vi "GenerateDefaultIBWFile.vi"(8 "error in (no error)":errorcluster) -> (0 "error out":errorcluster, 3 "Path":path)   [LabVIEW 2019]
uses:
  <vilib>/Utility/sysdir.llb/Get System Directory.vi
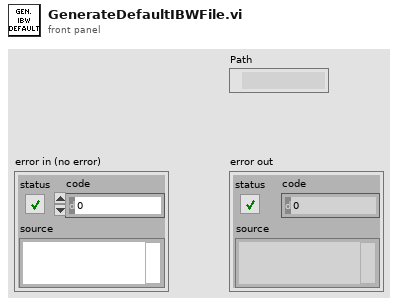
[diagram p1: front panel]
types:
  T1 = enum16{"open", "replace", "create", "open or create", "replace or create", "replace or create with confirmation"}
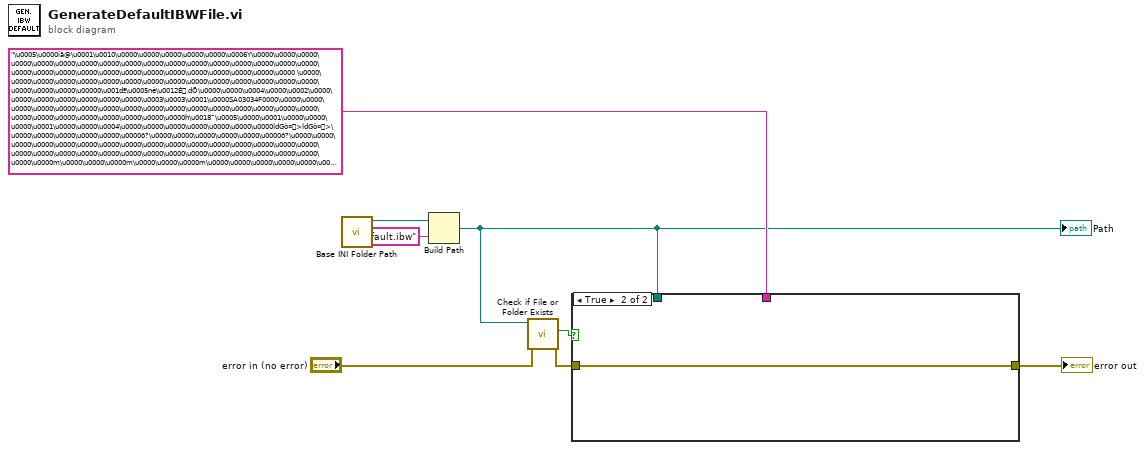
[diagram p0: block diagram]
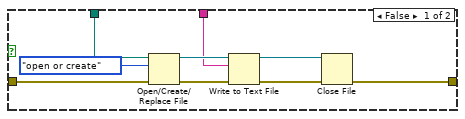
[diagram p2: hidden frame]
diagram:
  n1 = call "Base INI Folder Path.vi"() -> ("Base Path"=w8:path)  [unwired: 11 in]
  n2 = Build Path(base path=w8, name or relative path="Default.ibw") -> (appended path=w1:path)
  "Path" <- w1
  n3 = call <vilib>:"Check if File or Folder Exists.vi"("error in (no error)"="error in (no error)", "path"=w1) -> ("error out"=w3:errorcluster, "file or folder exists?"=w2:bool)  [unwired: 7 in, 1 out]
  n4 = case shown="True" w2 {
    tunnel: w1 -> [w17 _]
    tunnel: "\u0005\u0000îä@\u0001\u0010\u0000\u0000\u0000\u0000\u0000\u0006Y\u0000\u0000\u0000\u0000\u0000\u0000\u0000\u0000\u0000\u0000\u0000\u0000\u0000\u0000\u0000\u0000\u0000\u0000\u0000\u0000\u0000\u0000\u0000\u0000\u0000\u0000\u0000\u0000\u0000\u0000 \u0000\u0000\u0000\u0000\u0000\u0000\u0000\u0000\u0000\u0000\u0000\u0000\u0000\u0000\u0000\u0000\u0000\u0000\u00000\u001dª\u0005nè\u0012É.dÕ\u0000\u0000\u0004\u0000\u0002\u0000\u0000\u0000\u0000\u0000\u0000\u0000\u0003\u0003\u0001\u0000SA03034F0000\u0000\u0000\u0000\u0000\u0000\u0000\u0000\u0000\u0000\u0000\u0000\u0000\u0000\u0000\u0000\u0000\u0000\u0000\u0000\u0000\u0000\u0000\u0000\u0000h\u0018¯\u0005\u0000\u0001\u0000\u0000\u0000\u0001\u0000\u0000\u0004\u0000\u0000\u0000\u0000\u0000\u0000\u0000ÍdGò¤>ÍdGò¤>\u0000\u0000\u0000\u0000\u0000\u0000ð?\u0000\u0000\u0000\u0000\u0000\u0000ð?\u0000\u0000\u0000\u0000\u0000\u0000\u0000\u0000\u0000\u0000\u0000\u0000\u0000\u0000\u0000\u0000\u0000\u0000\u0000\u0000\u0000\u0000\u0000\u0000\u0000\u0000\u0000\u0000\u0000\u0000\u0000\u0000m\u0000\u0000\u0000m\u0000\u0000\u0000m\u0000\u0000\u0000\u0000\u0000\u0000\u0000\u0000\u0000\u0000\u0000\u0000\u0000\u0000\u0000\u0000\u0000\u0000\u0000\u0000\u0000\u0000\u0000\u0000\u0000\u0000\u0000\u0000\u0000\u0000\u0000\u0000\u0000\u0000\u0000\u0000\u0000\u0000\u0000\u0000\u0000\u0000\u0000\u0000\u0000\u0000\u0000\u0000\u0000\u0000\u0000\u0000\u0000\u0000\u0000\u0000\u0000\u0000\u0000H½t\u0013\u0000\u0000\u0000\u0000è¹t\u0013\u0002\u0000\u0003\u0000\u0003\u0000\u0000\u0000\u0000\u0000\u0000\u0000\u0000\u0000\u0000\u0000\u0000\u0000\u0000\u0000\u0000\u0000\u0000\u0000\u0000\u0000\u0000\u0000\u0000\u0000\u0000\u0000\u0000\u0000\u0000\u0000\u0000\u0000\u0000\u0000\u0000\u0000\u0000\u0000\u0000\u0000\u0000\u0000\u0000\u0000\u0000\u0000\u0000\u0000\u0000\u0000\u0000\u0000\u0000\u0000\u0000\u0000\u0000\u0000\u0003\u0000\u0001\u0000\u0001\u0000\u0000\u0000\u0000\u0000\u0000\u0000C\u0001\u0000\u0000b\u0001\u0000\u0000\u0000\u0000\u0000\u0000\u0000\u0000\u0000\u0000\u0000Àü.\u0000@±.\u0000À\u001b/\u0000@U/\u0000@/\u0000Àõ/\u0000`ÿ/\u0000ø\u00060\u0000x\b0\u0000àë/\u00000×/\u0000 ¡/\u0000 G/\u0000àÓ/\u0000p\u00050\u0000H'0\u0000ø\u001e0\u0000(:0\u0000 50\u0000\u0010\u00060\u0000\u0000ì/\u00000­/\u0000à/\u0000P/\u00000/\u0000°¿/\u0000 #/\u0000X\u00140\u0000@o/\u0000 û/\u0000àÚ/\u0000`Ò/\u0000 20\u0000 /\u0000\u0010¨0\u0000\u001f®\u0000C1\u0000Ôô1\u0000\u0003Ô2\u0000\u001d2\u0000@/\u0000\u001c0\u0000@®\u0000°11*\u000b2Öû2À\u001eª2\u0000v\u00161\u0000\u0000Ò¯\u0000êI±\u0000ñÆ±\u0000÷\u0011²\u0000E6²dI²..." ("data 2") -> [w13 _]
    tunnel: [w10 w18] -> w5
    tunnel: w3 -> [w9 w18]
    frame False {
      n5 = Open/Create/Replace File(file path (use dialog)=w17, error in=w9, operation (0:open)=T1."open or create") -> (refnum out=w15:refnum<file>, error out=w11:errorcluster)  [unwired: 3 in, 1 out]
      n6 = Write to Text File(file (use dialog)=w15, text=w13, error in=w11) -> (refnum out=w14:refnum<file>, error out=w12:errorcluster)  [unwired: 1 in, 1 out]
      n7 = Close File(refnum=w14, error in=w12) -> (error out=w10:errorcluster)  [unwired: 1 out]
    }
    frame True {
    }
  }
  "error out" <- w5
